vi "Scale Conversion.vi"(2 "y in":dbl, 3 "Convert Direction":u16(ring) items=["Nums to Pixels", "Pixel to Nums"], 4 "x in":dbl) -> (0 "y out":dbl, 1 "x out":dbl)   [LabVIEW 2012]
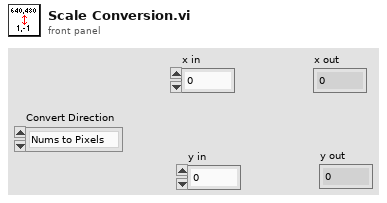
[diagram p1: front panel]
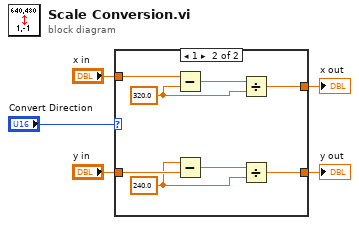
[diagram p0: block diagram]
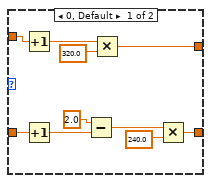
[diagram p2: hidden frame]
diagram:
  n1 = case shown="1" "Convert Direction" {
    tunnel: "y in" -> [w15 w23]
    tunnel: [w10 w20] -> w3
    tunnel: "x in" -> [w9 w19]
    tunnel: [w6 w16] -> w1
    frame 0, Default {
      n2 = Increment(x=w9) -> (x+1=w8:dbl)
      n3 = Increment(x=w15) -> (x+1=w13:dbl)
      n4 = Subtract(x=2.0, y=w13) -> (x-y=w12:dbl)
      n5 = Multiply(x=w8, y=320.0) -> (x*y=w6:dbl)
      n6 = Multiply(x=w12, y=240.0) -> (x*y=w10:dbl)
    }
    frame 1 {
      w17 = 320.0 ("y")
      w21 = 240.0 ("y")
      n7 = Subtract(x=w19, y=w17) -> (x-y=w18:dbl)
      n8 = Subtract(x=w21, y=w23) -> (x-y=w22:dbl)
      n9 = Divide(x=w18, y=w17) -> (x/y=w16:dbl)
      n10 = Divide(x=w22, y=w21) -> (x/y=w20:dbl)
    }
  }
  "x out" <- w1
  "y out" <- w3
